vi "Header or Footer polymorphic.vi"   [LabVIEW 2019]
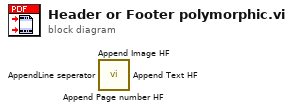
[diagram p0: block diagram]
diagram:
  n1 = call <userlib>:"Append Page number HF.vi"() -> ()  [unwired: 14 in, 2 out]
  n2 = call <userlib>:"Append Image HF.vi"() -> ()  [unwired: 14 in, 2 out]
  n3 = call <userlib>:"AppendLine seperator.vi"() -> ()  [unwired: 14 in, 2 out]
  n4 = call <userlib>:"Append Text HF.vi"() -> ()  [unwired: 14 in, 2 out]
